vi "Arduino Read Response.vi"(8 "error in":errorcluster, 11 "COM Port In":refnum<visa-resource-name>) -> (0 "error out":errorcluster, 2 "response":string, 3 "COM Port Out 2":refnum<visa-resource-name>)   [LabVIEW 2023, in "Arduino DAQ.lvlib"]
uses:
  Arduino DAQ.lvlib
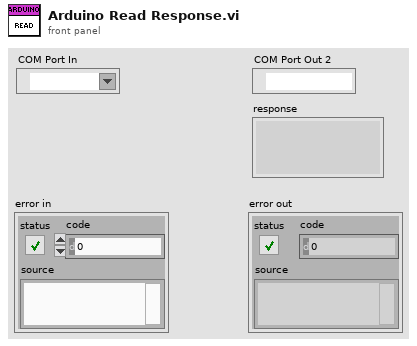
[diagram p1: front panel]
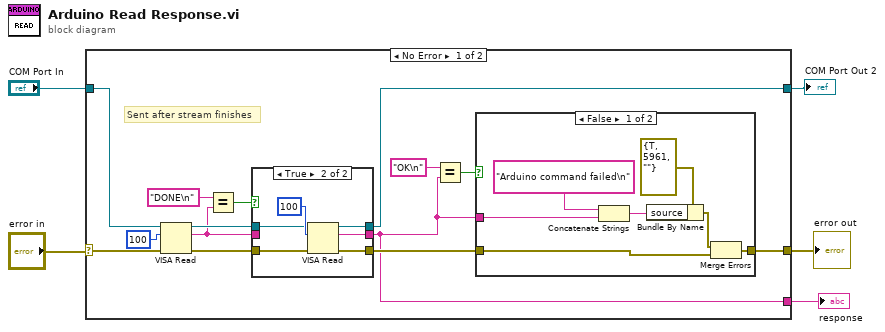
[diagram p0: block diagram]
diagram:
  n1 = case shown="No Error" "error in" {
    selector: "error in" -> [w15 w38]
    tunnel: [w17 w38] -> w5
    tunnel: "COM Port In" -> [w14 w37]
    tunnel: [w8 w37] -> w2
    tunnel: [w6 _] -> w1
    frame No Error {
      # "Sent after stream finishes"
      n2 = VISA Read(VISA resource name=w14, byte count=u32 100, error in (no error)=w15) -> (VISA resource name out=w11:refnum<visa-resource-name>, read buffer=w9:string, error out=w10:errorcluster)  [unwired: 1 out]
      n3 = Equal?(x="DONE\n" ("y"), y=w9) -> (x = y?=w12:bool)
      n4 = case shown="True" w12 {
        tunnel: w11 -> [w21 w26]
        tunnel: w10 -> [w20 w27]
        tunnel: [w21 w25] -> w8
        tunnel: [w20 w24] -> w7
        tunnel: [w22 w23] -> w6
        tunnel: w9 -> [w22 _]
        frame False {
        }
        frame True {
          n5 = VISA Read(VISA resource name=w26, byte count=u32 100, error in (no error)=w27) -> (VISA resource name out=w25:refnum<visa-resource-name>, read buffer=w23:string, error out=w24:errorcluster)  [unwired: 1 out]
        }
      }
      n6 = Equal?(x="OK\n" ("y"), y=w6) -> (x = y?=w18:bool)
      n7 = case shown="False" w18 {
        tunnel: [w35 w36] -> w17
        tunnel: w7 -> [w34 w36]
        tunnel: w6 -> [w30 _]
        frame False {
          n8 = Concatenate Strings("Arduino command failed\n" ("string"), w30) -> (w31:string)
          n9 = Bundle By Name(cluster=errorcluster {"status"=TRUE, "code"=5961, "source"=""} ("error constant"), "source"=w31) -> (w32:errorcluster)
          n10 = Merge Errors(w32, w34) -> (w35:errorcluster)
        }
        frame True {
        }
      }
    }
    frame Error {
    }
  }
  "error out" <- w5
  "COM Port Out 2" <- w2
  "response" <- w1
